vi "tsdb_load_lin_db.vi"(8 "error in (no error)":errorcluster caption="错误输入（无错误）", 9 "ABindChannels":i32[](array[ring])=[0] items=["CHN1", "CHN2", "CHN3", "CHN4", "CHN5", "CHN6", "CHN7", "CHN8", "CHN9", "CHN10", "CHN11", "CHN12", "CHN13", "CHN14", "CHN15", "CHN16", "CHN17", "CHN18", "CHN19", "CHN20", "CHN21", "CHN22", "CHN23", "CHN24", "CHN25", "CHN26", "CHN27", "CHN28", "CHN29", "CHN30", "CHN31", "CHN32"], 10 "ADBCAbsolutePath":path=path "C:/Users/DYR/Desktop/M110.dbc", 11 "路径输入":path) -> (0 "error out":errorcluster caption="错误输出", 1 "AId out":u32, 2 "function return":i32, 3 "路径输出":path)   [LabVIEW 2014]
doc: "Function Introduction ：\nLoad Lin database\nCall location ：\ninput parameter ：\nADBCAbsolute Path: DBC Absolute Path\nASupportedChannelsBed0: Supported Channels\nAfter successfully loading the database, the system returns the unique number assigned to the database\nReturn value ：\n==0: Execution successful\nOther values: Query error code"
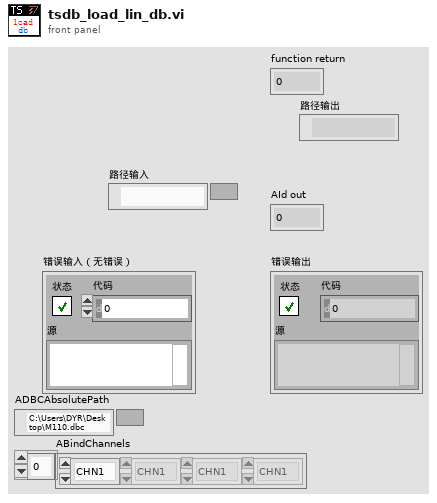
[diagram p1: front panel]
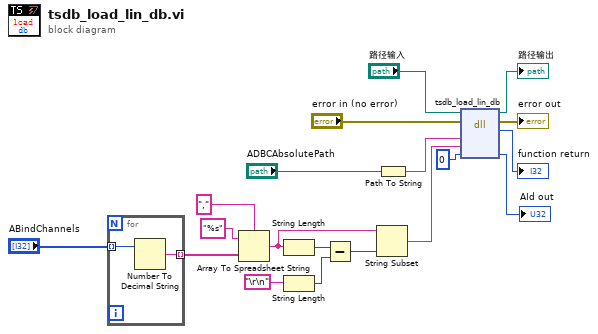
[diagram p0: block diagram]
diagram:
  n1 = for {
    tunnel: "ABindChannels" -> [w21] mode=indexing
    tunnel: [w20] -> w5 mode=indexing
    n2 = Number To Decimal String(number=w21) -> (decimal integer string=w20:string)  [unwired: 1 in]
  }
  n3 = Array To Spreadsheet String(delimiter (Tab)="," ("delimiter"), array=w5, 3:"%s" ("format string")) -> (spreadsheet string=w7:string)
  n4 = String Length(string=w7) -> (length=w9:i32)
  n5 = String Length(string="\r\n") -> (length=w8:i32)
  n6 = Subtract(x=w9, y=w8) -> (x-y=w6:i32)
  n7 = String Subset(string=w7, length (rest)=w6) -> (substring=w2:string)  [unwired: 1 in]
  n8 = Path To String(path="ADBCAbsolutePath") -> (string=w3:string)
  n9 = dll-call lib="D:/Work/LabVIEW Code/TSMaster Labview SDK/LabVIEW/LabVIEW-TSMasterAPI_CLN/TSMasterAPI_LabVIEW-2024-08-27 16-32-25/Not_organized_vi/TSMaster.*" fn="tsdb_load_lin_db"(path in="路径输入", error in="error in (no error)", "ALDF"=w3, "ASupportedChannelsBased0"=w2, "AId"=u32 0) -> (path out=→"路径输出":path, error out=→"error out":errorcluster, "return"=→"function return":i32, "AId"=→"AId out":u32)  [unwired: 3 in]
